vi "Check for Tone.vi"(6 "expected frequency (Hz)":dbl=-1.0, 8 "error in":errorcluster, 9 "window":T2=8 items=["None"=0, "Hanning"=1, "Hamming"=2, "Blackman-Harris"=3, "Exact Blackman"=4, "Blackman"=5, "Flat Top"=6, "4 Term B-Harris "=7, "7 Term B-Harris"=8, "Low Sidelobe"=9, "Force"=64, "Exponential"=65, "Blackman Nuttall"=11, "Triangle"=30, "Bartlett-Hanning"=31, "Bohman"=32, "Parzen"=33, "Welch"=34, "Kaiser"=60, "Dolph-Chebyshev"=61, "Gaussian"=62], 10 "frequency range":T1={"start frequency"=20.0, "stop frequency"=20000.0}, 11 "waveform":waveform(dbl)) -> (0 "error out":errorcluster, 2 "tone detected?":bool, 3 "frequency":dbl format="%#_g Hz")   [LabVIEW 2025, in "Tone Measurements.lvlib" / "Tone Measurements.lvclass"]
uses:
  Tone Measurements.lvclass
  <vilib>/addons/_NISVFA/_Shared subVIs/Controls/svc_Window.ctl
  <vilib>/addons/_NISVFA/_Spectrum Processing/SVFA Power in Band (1 Ch).vi
  <vilib>/addons/_NISVFA/_Spectrum Processing/SVFA Spectrum Peak Search (1 Ch).vi
  <vilib>/addons/_NISVFA/_Spectrum Processing/SVFA Get Spectrum Subset.vi
  <vilib>/addons/_NISVFA/_Spectrum Processing/SVFA Get Spectrum Subset (1 Ch).vi
  <vilib>/addons/_NISVFA/_Shared subVIs/Common/svc_Window Parameters.vi
  <vilib>/addons/_NISVFA/_Shared subVIs/Common/svc_Spectrum Units.vi
  <vilib>/addons/_NISVFA/_Spectrum Processing/SVFA Unit Conversion.vi
  <vilib>/addons/_NISVFA/_Spectrum Processing/SVFA Unit Conversion (1 Ch).vi
  <vilib>/addons/_NISVFA/_Spectrum Processing/subVIs/svfa_Spectrum Info Window to windowTd Type Def.vi
  <vilib>/addons/_NISVFA/_Spectrum Processing/subVIs/svfa_Spectrum Peak Search.vi
  <vilib>/addons/_NISVFA/_Shared subVIs/Common/svc_Build Unit Label for Frequency Range.vi
  <vilib>/addons/_NISVFA/_Shared subVIs/Common/svc_Check Frequency Range in Spectrum.vi
  <vilib>/addons/_NISVFA/_Shared subVIs/Common/svc_Format Value (DBL).vi
  <vilib>/addons/_NISVFA/_Shared subVIs/Common/svc_Get Weighting Enum and Labels.vi
  <vilib>/addons/_NISVFA/_Shared subVIs/Common/svc_Engineering Units to Unit Label.vi
  <vilib>/addons/_NISVFA/_Shared subVIs/Common/svc_Surround NonAlpha String with Parentheses.vi
  <vilib>/dlg_ctls.llb/Space Constant.vi
  <vilib>/addons/_NISVFA/_Spectrum Processing/subVIs/svfa_Conversion Utility (spectrum info).vi
  <vilib>/addons/_NISVFA/_Spectrum Processing/subVIs/svfa_Peak Rough Search Indices.vi
  <vilib>/addons/_NISVFA/_Shared subVIs/Common/svc_Check Frequency Range in Bandwidth.vi
  <vilib>/addons/_NISVFA/_Shared subVIs/Common/svc_Convert Start and Stop to Start Index and Length.vi
  <vilib>/addons/_NISVFA/_Shared subVIs/Common/svc_Unit Label Lexical Class.vi
  <vilib>/addons/_NISVFA/_Spectrum Processing/subVIs/svfa_Peak to RMS to Peak2Peak.vi
  <vilib>/addons/_NISVFA/_Spectrum Processing/subVIs/svfa_Mag to Mag2.vi
  <vilib>/addons/_NISVFA/_Spectrum Processing/subVIs/svfa_Linear to dB.vi
  <vilib>/addons/_NISVFA/_Spectrum Processing/subVIs/svfa_dBrefA to dBrefB.vi
  <vilib>/addons/_NISVFA/_Spectrum Processing/subVIs/svfa_Spectrum to Spectral Density.vi
  <vilib>/addons/_NISVFA/_Subset FFT/SVFA Power Spectrum Subset (1 Ch).vi
  <vilib>/addons/_NISVFA/_Spectrum Processing/subVIs/svfa_Three Finger Peak Search.vi
  <vilib>/addons/_NISVFA/_Shared subVIs/Common/svc_Caller VI Returned in Error Source.vi
  <vilib>/addons/_NISVFA/_Shared subVIs/Common/svc_Convert Frequency to Frequency String.vi
  <vilib>/Analysis/4window.llb/window parameters.vi
  <vilib>/Analysis/4window.llb/Window Properties.vi
  <vilib>/Analysis/4window.llb/Window Properties by Name.vi
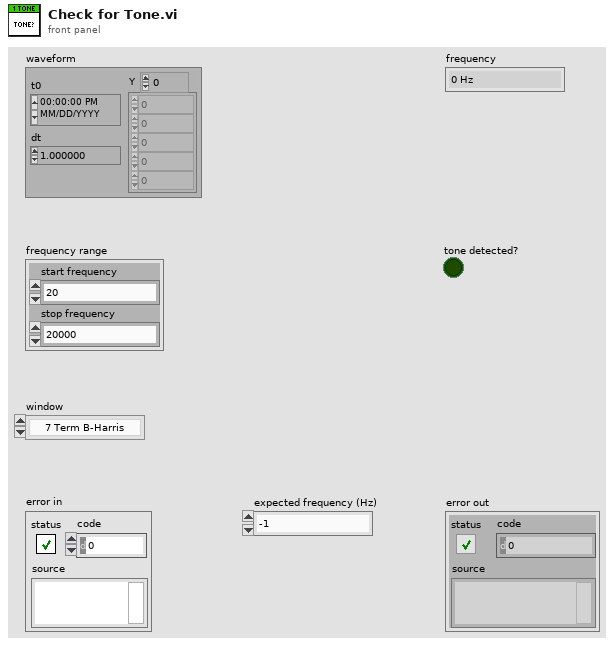
[diagram p1: front panel]
types:
  T1 = cluster{"start frequency":dbl, "stop frequency":dbl}
  T2 = typedef "svc_Window.ctl" = u32
  T3 = cluster{"single/multiple":enum16{"Multiple Peaks", "Single Max Peak"}, "threshold":dbl}
  T4 = typedef "svc_Spectrum Info.ctl" = cluster{"channel name":string, "description":string, "x-axis units":T5, "spectral info":cluster{"spectrum type":T6, "linear/dB":enum16{"linear", "dB"}, "window":u16, "window size":i32, "FFT size":i32}, "engineering units":T7, "custom label":string, "dB reference [EU]":dbl, "peak units":enum16{"rms", "peak", "peak-peak"}, "weighting filter":T8, "spectral density?":bool, "unit label":string, "spectrum skewed?":bool, "complimentary spectrum units":T9}
  T5 = typedef "svc_X-Axis Units.ctl" = u16
  T6 = typedef "svc_Spectrum Type.ctl" = enum16{"FFT Spectrum [complex]", "Amplitude [Magnitude]", "Power [Magnitude^2]", "Cross Spectrum [complex]", "Frequency Response [Complex]"}
  T7 = typedef "svc_Engineering Units Text Ring.ctl" = u16
  T8 = typedef "svc_Weighting Filter Text Ring.ctl" = u16
  T9 = typedef "svc_Complimentary Spectrum Units.ctl" = enum16{"none", "radians", "degrees", "cycles", "imaginary"}
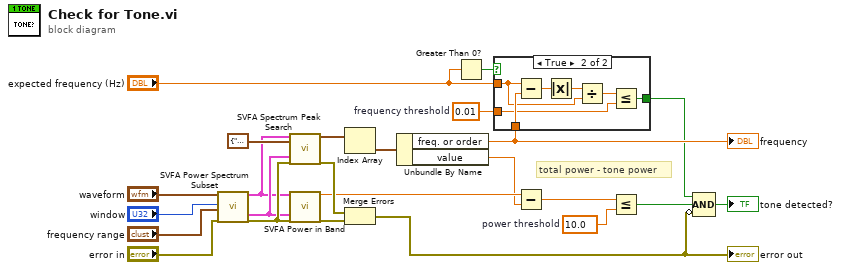
[diagram p0: block diagram]
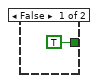
[diagram p2: hidden frame]
diagram:
  w5 = 0.01  # frequency threshold
  w9 = 10.0  # power threshold
  # "total power - tone power"
  n1 = call-poly <vilib>:"SVFA Power Spectrum Subset.vi"("scaled signal [EU]"="waveform", "window"="window", "frequency range"="frequency range", "error in (no error)"="error in") -> ("power spectrum [dB EU]"=w19:cluster{"f0":dbl, "df":dbl, "magnitude":dbl[]}, "spectrum info"=w20:T4, "error out"=w21:errorcluster)  [unwired: 10 in, 3 out]
  n2 = call-poly <vilib>:"SVFA Spectrum Peak Search.vi"("spectrum"=w19, "peak search settings"=T3 {"single/multiple"=enum."Single Max Peak", "threshold"=inf}, "spectrum info in"=w20, "error in (no error)"=w21) -> ("peaks"=w23:cluster{"freq. or order":dbl, "value":dbl}[], "error out"=w15:errorcluster)  [unwired: 11 in, 3 out]
  n3 = call-poly <vilib>:"SVFA Power in Band.vi"("spectrum"=w19, "spectrum info"=w20, "error in (no error)"=w21) -> ("power in band"=w12:dbl, "error out"=w14:errorcluster)  [unwired: 14 in, 1 out]
  n4 = Index Array(array=w23) -> (element=w24:cluster{"freq. or order":dbl, "value":dbl})  [unwired: 1 in]
  n5 = Merge Errors(w15, w14) -> (w1:errorcluster)
  "error out" <- w1
  n6 = Unbundle By Name(w24) -> ("freq. or order"=w7:dbl, "value"=w11:dbl)
  "frequency" <- w7
  n7 = Greater Than 0?(x="expected frequency (Hz)") -> (x > 0?=w6:bool)
  n8 = case shown="True" w6 {
    tunnel: "expected frequency (Hz)" -> [_ w30]
    tunnel: w7 -> [_ w32]
    tunnel: w5 -> [_ w28]
    tunnel: [TRUE w27] -> w3
    frame False {
    }
    frame True {
      n9 = Subtract(x=w30, y=w32) -> (x-y=w31:dbl)
      n10 = Absolute Value(x=w31) -> (abs(x)=w26:dbl)
      n11 = Divide(x=w26, y=w30) -> (x/y=w29:dbl)
      n12 = Less Or Equal?(x=w29, y=w28) -> (x <= y?=w27:bool)
    }
  }
  n13 = Subtract(x=w12, y=w11) -> (x-y=w10:dbl)
  n14 = Less Or Equal?(x=w10, y=w9) -> (x <= y?=w4:bool)
  n15 = Compound Arithmetic op=AND(w3, w4, invert w1) -> (→"tone detected?":bool)
